vi "Game_Init.vi"(8 "error in (no error)":errorcluster) -> (0 "error out":errorcluster, 2 "Players array":T1[](array[typedef]), 3 "Queue Bus OUT":T2)   [LabVIEW 2020]
uses:
  Typedefs/queueBus.ctl
  Typedefs/communicationData.ctl
  Typedefs/game_player.ctl
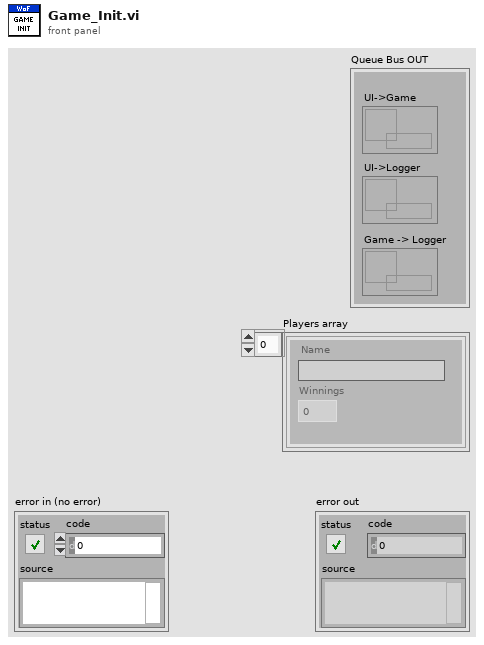
[diagram p1: front panel]
types:
  T1 = typedef "game_player.ctl" = cluster{"Name":string, "Winnings":dbl}
  T2 = typedef "queueBus.ctl" = cluster{"UI->Game":refnum<queue>, "UI->Logger":refnum<queue>, "Game -> Logger":refnum<queue>}
  T3 = typedef "communicationData.ctl" = cluster{"command":string, "payload":variant, "response":variant}
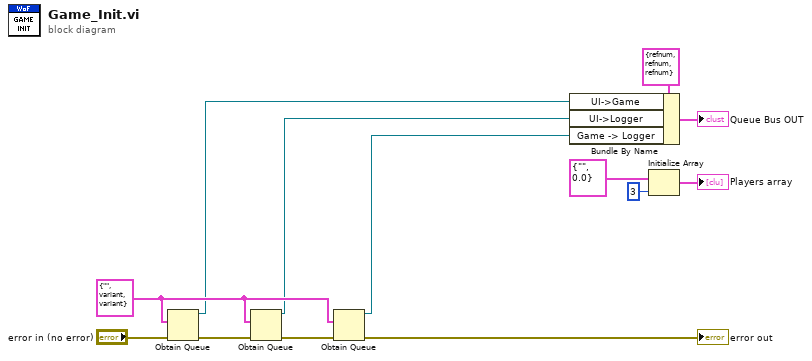
[diagram p0: block diagram]
diagram:
  w7 = T3 {"command"="", "payload"=variant, "response"=variant} ("communication")
  n1 = Obtain Queue(element data type=w7, error in (no error)="error in (no error)") -> (queue out=w4:refnum<queue>, error out=w12:errorcluster)  [unwired: 3 in, 1 out]
  n2 = Obtain Queue(element data type=w7, error in (no error)=w12) -> (queue out=w6:refnum<queue>, error out=w9:errorcluster)  [unwired: 3 in, 1 out]
  n3 = Obtain Queue(element data type=w7, error in (no error)=w9) -> (queue out=w5:refnum<queue>, error out=→"error out":errorcluster)  [unwired: 3 in, 1 out]
  n4 = Bundle By Name(cluster=T2 {"UI->Game"=refnum, "UI->Logger"=refnum, "Game -> Logger"=refnum} ("Queue Bus"), "UI->Game"=w4, "UI->Logger"=w6, "Game -> Logger"=w5) -> (→"Queue Bus OUT":T2)
  n5 = Initialize Array(T1 {"Name"="", "Winnings"=0.0} ("Player"), 3 ("dimension size")) -> (→"Players array":T1[])
